vi "大富翁.vi"() -> ()   [LabVIEW 2014] (continued)
                n1038 = call "顏色轉數字.vi"("顏色數字"=w422) -> ("數字"=w425:dbl)  [unwired: 2 in]
                n1039 = case shown="1, Default" w425 {
                  tunnel: [w443 w444 w445 w446] -> w429
                  frame 1, Default {
                    n1040 = local read "玩家一財產"() -> (w443:dbl)
                  }
                  frame 2 {
                    n1041 = local read "玩家二財產"() -> (w444:dbl)
                  }
                  frame 3 {
                    n1042 = local read "玩家三財產"() -> (w445:dbl)
                  }
                  frame 4 {
                    n1043 = local read "玩家四財產"() -> (w446:dbl)
                  }
                }
                n1044 = call "走到地.vi"("房子數量"=w436, "自己的地?"=w437, "旅館數量"=w435, "編號"=w434, "走到人財產"=w433) -> ("走到人-?"=w432:dbl, "蓋第幾棟"=w430:dbl, "地主+?"=w428:dbl, "破產?"=w424:bool)
                n1045 = Subtract(x=w433, y=w432) -> (x-y=w431:dbl)
                n1046 = Add(x=w428, y=w429) -> (x+y=w426:dbl)
                n1047 = case shown="1, Default" w425 {
                  tunnel: w426 -> [w439 w440 w441 w442]
                  frame 1, Default {
                    n1048 = local write "玩家一財產"(w439) -> ()
                  }
                  frame 2 {
                    n1049 = local write "玩家二財產"(w440) -> ()
                  }
                  frame 3 {
                    n1050 = local write "玩家三財產"(w441) -> ()
                  }
                  frame 4 {
                    n1051 = local write "玩家四財產"(w442) -> ()
                  }
                }
                n1052 = case shown="8" w430 {
                  frame 0, Default {
                  }
                  frame 1 {
                    n1053 = flat-sequence {
                      frame #0 {
                        n1054 = local write "3房1"(TRUE ("1房1")) -> ()
                      }
                      frame #1 {
                        n1055 = property on="3房1" class="Bool (strict)"("Visible"=TRUE) -> ()  [unwired: 2 in, 2 out]
                      }
                    }
                  }
                  frame 2 {
                    n1056 = flat-sequence {
                      frame #0 {
                        n1057 = local write "3房2"(TRUE ("1房2")) -> ()
                      }
                      frame #1 {
                        n1058 = property on="3房2" class="Bool (strict)"("Visible"=TRUE ("1房2")) -> ()  [unwired: 2 in, 2 out]
                      }
                    }
                  }
                  frame 3 {
                    n1059 = flat-sequence {
                      frame #0 {
                        n1060 = local write "3房3"(TRUE) -> ()
                      }
                      frame #1 {
                        n1061 = property on="3房3" class="Bool (strict)"("Visible"=TRUE) -> ()  [unwired: 2 in, 2 out]
                      }
                    }
                  }
                  frame 4 {
                    n1062 = flat-sequence {
                      frame #0 {
                        n1063 = local write "3房4"(TRUE) -> ()
                      }
                      frame #1 {
                        n1064 = property on="3房4" class="Bool (strict)"("Visible"=TRUE) -> ()  [unwired: 2 in, 2 out]
                      }
                    }
                  }
                  frame 5 {
                    n1065 = flat-sequence {
                      frame #0 {
                        n1066 = local write "3旅1"(TRUE) -> ()
                      }
                      frame #1 {
                        n1067 = property on="3旅1" class="Bool (strict)"("Visible"=TRUE) -> ()  [unwired: 2 in, 2 out]
                      }
                    }
                  }
                  frame 6 {
                    n1068 = flat-sequence {
                      frame #0 {
                        n1069 = local write "3旅2"(TRUE) -> ()
                      }
                      frame #1 {
                        n1070 = property on="3旅2" class="Bool (strict)"("Visible"=TRUE) -> ()  [unwired: 2 in, 2 out]
                      }
                    }
                  }
                  frame 7 {
                    n1071 = flat-sequence {
                      frame #0 {
                        n1072 = local write "3旅3"(TRUE) -> ()
                      }
                      frame #1 {
                        n1073 = property on="3旅3" class="Bool (strict)"("Visible"=TRUE) -> ()  [unwired: 2 in, 2 out]
                      }
                    }
                  }
                  frame 8 {
                    n1074 = flat-sequence {
                      frame #0 {
                        n1075 = local write "3旅4"(TRUE) -> ()
                      }
                      frame #1 {
                        n1076 = property on="3旅4" class="Bool (strict)"("Visible"=TRUE) -> ()  [unwired: 2 in, 2 out]
                      }
                    }
                  }
                }
                n1077 = case shown="1, Default" w427 {
                  tunnel: w431 -> [w463 w464 w465 w466]
                  frame 1, Default {
                    n1078 = local write "玩家一財產"(w463) -> ()
                  }
                  frame 2 {
                    n1079 = local write "玩家二財產"(w464) -> ()
                  }
                  frame 3 {
                    n1080 = local write "玩家三財產"(w465) -> ()
                  }
                  frame 4 {
                    n1081 = local write "玩家四財產"(w466) -> ()
                  }
                }
              }
              frame True {
                # "無主地"
                n1082 = call "購買土地.vi"() -> ("確定 2"=w473:bool)  [unwired: 3 in]
                n1083 = case shown="True" w473 {
                  tunnel: w472 -> [_ w477]
                  frame False {
                    # "不買"
                  }
                  frame True {
                    # "要買"
                    n1084 = local read "換誰?"() -> (w478:dbl)
                    n1085 = case shown="4" w478 {
                      tunnel: [w505 w506 w507 w508] -> w476
                      frame 1, Default {
                        n1086 = local read "玩家一財產"() -> (w505:dbl)
                      }
                      frame 2 {
                        n1087 = local read "玩家二財產"() -> (w506:dbl)
                      }
                      frame 3 {
                        n1088 = local read "玩家三財產"() -> (w507:dbl)
                      }
                      frame 4 {
                        n1089 = local read "玩家四財產"() -> (w508:dbl)
                      }
                    }
                    n1090 = call "各種價格.vi"("Numeric"=w477) -> ("買空地"=w475:dbl)  [unwired: 4 in, 5 out]
                    n1091 = Greater Or Equal?(x=w476, y=w475) -> (x >= y?=w474:bool)
                    n1092 = case shown="True" w474 {
                      tunnel: w477 -> [_ w479]
                      frame False {
                        # "錢不夠"
                        n1093 = call "錢不夠.vi"() -> ()  [unwired: 4 in]
                      }
                      frame True {
                        # "錢夠"
                        n1094 = local read "換誰?"() -> (w480:dbl)
                        n1095 = case shown="3" w480 {
                          selector: w480 -> [w484 w490 w496 w502]
                          tunnel: w479 -> [w483 w489 w495 w501]
                          frame 1, Default {
                            # "誰買了地"
                            n1096 = call "各種價格.vi"("Numeric"=w483) -> ("買空地"=w482:dbl)  [unwired: 4 in, 5 out]
                            n1097 = local read "玩家一財產"() -> (w486:dbl)
                            n1098 = Subtract(x=w486, y=w482) -> (x-y=w485:dbl)
                            n1099 = local write "玩家一財產"(w485) -> ()
                            n1100 = call "數字轉顏色.vi"("數字"=w484) -> ("顏色數字"=w481:dbl)  [unwired: 2 in]
                            n1101 = local write "3台北市"(w481) -> ()
                            n1102 = local write "台北市所有"(w481) -> ()
                          }
                          frame 2 {
                            # "誰買了地"
                            n1103 = call "各種價格.vi"("Numeric"=w489) -> ("買空地"=w488:dbl)  [unwired: 4 in, 5 out]
                            n1104 = local read "玩家二財產"() -> (w492:dbl)
                            n1105 = Subtract(x=w492, y=w488) -> (x-y=w491:dbl)
                            n1106 = local write "玩家二財產"(w491) -> ()
                            n1107 = call "數字轉顏色.vi"("數字"=w490) -> ("顏色數字"=w487:dbl)  [unwired: 2 in]
                            n1108 = local write "3台北市"(w487) -> ()
                            n1109 = local write "台北市所有"(w487) -> ()
                          }
                          frame 3 {
                            # "誰買了地"
                            n1110 = local read "玩家三財產"() -> (w497:dbl)
                            n1111 = call "各種價格.vi"("Numeric"=w495) -> ("買空地"=w494:dbl)  [unwired: 4 in, 5 out]
                            n1112 = Subtract(x=w497, y=w494) -> (x-y=w498:dbl)
                            n1113 = call "數字轉顏色.vi"("數字"=w496) -> ("顏色數字"=w493:dbl)  [unwired: 2 in]
                            n1114 = local write "玩家三財產"(w498) -> ()
                            n1115 = local write "3台北市"(w493) -> ()
                            n1116 = local write "台北市所有"(w493) -> ()
                          }
                          frame 4 {
                            # "誰買了地"
                            n1117 = call "各種價格.vi"("Numeric"=w501) -> ("買空地"=w500:dbl)  [unwired: 4 in, 5 out]
                            n1118 = local read "玩家四財產"() -> (w504:dbl)
                            n1119 = Subtract(x=w504, y=w500) -> (x-y=w503:dbl)
                            n1120 = local write "玩家四財產"(w503) -> ()
                            n1121 = call "數字轉顏色.vi"("數字"=w502) -> ("顏色數字"=w499:dbl)  [unwired: 2 in]
                            n1122 = local write "3台北市"(w499) -> ()
                            n1123 = local write "台北市所有"(w499) -> ()
                          }
                        }
                      }
                    }
                  }
                }
              }
            }
          }
          frame 4 {
            n1124 = local read "基隆市所有"() -> (w509:u32)
            n1125 = Equal?(x=w509, y=u32 16777215) -> (x = y?=w512:bool)
            n1126 = case shown="True" w512 {
              tunnel: w511 -> [w535 w573]
              tunnel: [w525 FALSE] -> w510
              frame False {
                # "有主地"
                n1127 = local read "換誰?"() -> (w528:dbl)
                n1128 = local read "基隆市所有"() -> (w516:u32)
                n1129 = call "數字轉顏色.vi"("數字"=w528) -> ("顏色數字"=w539:dbl)  [unwired: 2 in]
                n1130 = case shown="4" w528 {
                  tunnel: [w568 w569 w570 w571] -> w534
                  frame 1, Default {
                    n1131 = local read "玩家一財產"() -> (w568:dbl)
                  }
                  frame 2 {
                    n1132 = local read "玩家二財產"() -> (w569:dbl)
                  }
                  frame 3 {
                    n1133 = local read "玩家三財產"() -> (w570:dbl)
                  }
                  frame 4 {
                    n1134 = local read "玩家四財產"() -> (w571:dbl)
                  }
                }
                n1135 = Equal?(x=w516, y=w539) -> (x = y?=w538:bool)
                n1136 = local read "基隆市所有"() -> (w515:u32)
                n1137 = local read "4旅4"() -> (w517:bool)
                n1138 = local read "4旅3"() -> (w518:bool)
                n1139 = local read "4旅2"() -> (w519:bool)
                n1140 = local read "4旅1"() -> (w520:bool)
                n1141 = local read "4房4"() -> (w521:bool)
                n1142 = local read "4房3"() -> (w522:bool)
                n1143 = local read "4房2"() -> (w523:bool)
                n1144 = local read "4房1"() -> (w524:bool)
                n1145 = call "房子數量.vi"("房子 1"=w524, "房子 2"=w523, "房子 3"=w522, "房子 4"=w521, "旅館 1"=w520, "旅館 2"=w519, "旅館 3"=w518, "旅館 4"=w517) -> ("房子數"=w537:dbl, "旅館數"=w536:dbl)  [unwired: 18 in]
                n1146 = call "顏色轉數字.vi"("顏色數字"=w515) -> ("數字"=w526:dbl)  [unwired: 2 in]
                n1147 = case shown="1, Default" w526 {
                  tunnel: [w544 w545 w546 w547] -> w530
                  frame 1, Default {
                    n1148 = local read "玩家一財產"() -> (w544:dbl)
                  }
                  frame 2 {
                    n1149 = local read "玩家二財產"() -> (w545:dbl)
                  }
                  frame 3 {
                    n1150 = local read "玩家三財產"() -> (w546:dbl)
                  }
                  frame 4 {
                    n1151 = local read "玩家四財產"() -> (w547:dbl)
                  }
                }
                n1152 = call "走到地.vi"("房子數量"=w537, "自己的地?"=w538, "旅館數量"=w536, "編號"=w535, "走到人財產"=w534) -> ("走到人-?"=w533:dbl, "蓋第幾棟"=w531:dbl, "地主+?"=w529:dbl, "破產?"=w525:bool)
                n1153 = Subtract(x=w534, y=w533) -> (x-y=w532:dbl)
                n1154 = Add(x=w529, y=w530) -> (x+y=w527:dbl)
                n1155 = case shown="1, Default" w526 {
                  tunnel: w527 -> [w540 w541 w542 w543]
                  frame 1, Default {
                    n1156 = local write "玩家一財產"(w540) -> ()
                  }
                  frame 2 {
                    n1157 = local write "玩家二財產"(w541) -> ()
                  }
                  frame 3 {
                    n1158 = local write "玩家三財產"(w542) -> ()
                  }
                  frame 4 {
                    n1159 = local write "玩家四財產"(w543) -> ()
                  }
                }
                n1160 = case shown="8" w531 {
                  frame 0, Default {
                  }
                  frame 1 {
                    n1161 = flat-sequence {
                      frame #0 {
                        n1162 = local write "4房1"(TRUE ("1房1")) -> ()
                      }
                      frame #1 {
                        n1163 = property on="4房1" class="Bool (strict)"("Visible"=TRUE) -> ()  [unwired: 2 in, 2 out]
                      }
                    }
                  }
                  frame 2 {
                    n1164 = flat-sequence {
                      frame #0 {
                        n1165 = local write "4房2"(TRUE ("1房2")) -> ()
                      }
                      frame #1 {
                        n1166 = property on="4房2" class="Bool (strict)"("Visible"=TRUE ("1房2")) -> ()  [unwired: 2 in, 2 out]
                      }
                    }
                  }
                  frame 3 {
                    n1167 = flat-sequence {
                      frame #0 {
                        n1168 = local write "4房3"(TRUE) -> ()
                      }
                      frame #1 {
                        n1169 = property on="4房3" class="Bool (strict)"("Visible"=TRUE) -> ()  [unwired: 2 in, 2 out]
                      }
                    }
                  }
                  frame 4 {
                    n1170 = flat-sequence {
                      frame #0 {
                        n1171 = local write "4房4"(TRUE) -> ()
                      }
                      frame #1 {
                        n1172 = property on="4房4" class="Bool (strict)"("Visible"=TRUE) -> ()  [unwired: 2 in, 2 out]
                      }
                    }
                  }
                  frame 5 {
                    n1173 = flat-sequence {
                      frame #0 {
                        n1174 = local write "4旅1"(TRUE) -> ()
                      }
                      frame #1 {
                        n1175 = property on="4旅1" class="Bool (strict)"("Visible"=TRUE) -> ()  [unwired: 2 in, 2 out]
                      }
                    }
                  }
                  frame 6 {
                    n1176 = flat-sequence {
                      frame #0 {
                        n1177 = local write "4旅2"(TRUE) -> ()
                      }
                      frame #1 {
                        n1178 = property on="4旅2" class="Bool (strict)"("Visible"=TRUE) -> ()  [unwired: 2 in, 2 out]
                      }
                    }
                  }
                  frame 7 {
                    n1179 = flat-sequence {
                      frame #0 {
                        n1180 = local write "4旅3"(TRUE) -> ()
                      }
                      frame #1 {
                        n1181 = property on="4旅3" class="Bool (strict)"("Visible"=TRUE) -> ()  [unwired: 2 in, 2 out]
                      }
                    }
                  }
                  frame 8 {
                    n1182 = flat-sequence {
                      frame #0 {
                        n1183 = local write "4旅4"(TRUE) -> ()
                      }
                      frame #1 {
                        n1184 = property on="4旅4" class="Bool (strict)"("Visible"=TRUE) -> ()  [unwired: 2 in, 2 out]
                      }
                    }
                  }
                }
                n1185 = case shown="1, Default" w528 {
                  tunnel: w532 -> [w564 w565 w566 w567]
                  frame 1, Default {
                    n1186 = local write "玩家一財產"(w564) -> ()
                  }
                  frame 2 {
                    n1187 = local write "玩家二財產"(w565) -> ()
                  }
                  frame 3 {
                    n1188 = local write "玩家三財產"(w566) -> ()
                  }
                  frame 4 {
                    n1189 = local write "玩家四財產"(w567) -> ()
                  }
                }
              }
              frame True {
                # "無主地"
                n1190 = call "購買土地.vi"() -> ("確定 2"=w574:bool)  [unwired: 3 in]
                n1191 = case shown="True" w574 {
                  tunnel: w573 -> [_ w578]
                  frame False {
                    # "不買"
                  }
                  frame True {
                    # "要買"
                    n1192 = local read "換誰?"() -> (w579:dbl)
                    n1193 = case shown="4" w579 {
                      tunnel: [w606 w607 w608 w609] -> w577
                      frame 1, Default {
                        n1194 = local read "玩家一財產"() -> (w606:dbl)
                      }
                      frame 2 {
                        n1195 = local read "玩家二財產"() -> (w607:dbl)
                      }
                      frame 3 {
                        n1196 = local read "玩家三財產"() -> (w608:dbl)
                      }
                      frame 4 {
                        n1197 = local read "玩家四財產"() -> (w609:dbl)
                      }
                    }
                    n1198 = call "各種價格.vi"("Numeric"=w578) -> ("買空地"=w576:dbl)  [unwired: 4 in, 5 out]
                    n1199 = Greater Or Equal?(x=w577, y=w576) -> (x >= y?=w575:bool)
                    n1200 = case shown="True" w575 {
                      tunnel: w578 -> [_ w580]
                      frame False {
                        # "錢不夠"
                        n1201 = call "錢不夠.vi"() -> ()  [unwired: 4 in]
                      }
                      frame True {
                        # "錢夠"
                        n1202 = local read "換誰?"() -> (w581:dbl)
                        n1203 = case shown="4" w581 {
                          selector: w581 -> [w585 w591 w597 w603]
                          tunnel: w580 -> [w584 w590 w596 w602]
                          frame 1, Default {
                            # "誰買了地"
                            n1204 = call "各種價格.vi"("Numeric"=w584) -> ("買空地"=w583:dbl)  [unwired: 4 in, 5 out]
                            n1205 = local read "玩家一財產"() -> (w587:dbl)
                            n1206 = Subtract(x=w587, y=w583) -> (x-y=w586:dbl)
                            n1207 = local write "玩家一財產"(w586) -> ()
                            n1208 = call "數字轉顏色.vi"("數字"=w585) -> ("顏色數字"=w582:dbl)  [unwired: 2 in]
                            n1209 = local write "4基隆市"(w582) -> ()
                            n1210 = local write "基隆市所有"(w582) -> ()
                          }
                          frame 2 {
                            # "誰買了地"
                            n1211 = call "各種價格.vi"("Numeric"=w590) -> ("買空地"=w589:dbl)  [unwired: 4 in, 5 out]
                            n1212 = local read "玩家二財產"() -> (w593:dbl)
                            n1213 = Subtract(x=w593, y=w589) -> (x-y=w592:dbl)
                            n1214 = local write "玩家二財產"(w592) -> ()
                            n1215 = call "數字轉顏色.vi"("數字"=w591) -> ("顏色數字"=w588:dbl)  [unwired: 2 in]
                            n1216 = local write "4基隆市"(w588) -> ()
                            n1217 = local write "基隆市所有"(w588) -> ()
                          }
                          frame 3 {
                            # "誰買了地"
                            n1218 = local read "玩家三財產"() -> (w598:dbl)
                            n1219 = call "各種價格.vi"("Numeric"=w596) -> ("買空地"=w595:dbl)  [unwired: 4 in, 5 out]
                            n1220 = Subtract(x=w598, y=w595) -> (x-y=w599:dbl)
                            n1221 = call "數字轉顏色.vi"("數字"=w597) -> ("顏色數字"=w594:dbl)  [unwired: 2 in]
                            n1222 = local write "玩家三財產"(w599) -> ()
                            n1223 = local write "4基隆市"(w594) -> ()
                            n1224 = local write "基隆市所有"(w594) -> ()
                          }
                          frame 4 {
                            # "誰買了地"
                            n1225 = call "各種價格.vi"("Numeric"=w602) -> ("買空地"=w601:dbl)  [unwired: 4 in, 5 out]
                            n1226 = local read "玩家四財產"() -> (w605:dbl)
                            n1227 = Subtract(x=w605, y=w601) -> (x-y=w604:dbl)
                            n1228 = local write "玩家四財產"(w604) -> ()
                            n1229 = call "數字轉顏色.vi"("數字"=w603) -> ("顏色數字"=w600:dbl)  [unwired: 2 in]
                            n1230 = local write "4基隆市"(w600) -> ()
                            n1231 = local write "基隆市所有"(w600) -> ()
                          }
                        }
                      }
                    }
                  }
                }
              }
            }
          }
          frame 5, 16, 28 {
            # "命運"
            n1232 = local read "白色恐怖?"() -> (w611:bool)
            n1233 = case shown="False" w611 {
              tunnel: [w613 FALSE] -> w610
              frame False {
                # "非白色恐怖"
                n1234 = Random Number (0-1)() -> (number: 0 to 1=w618:dbl)
                n1235 = Multiply(x=w618, y=100.0) -> (x*y=w614:dbl)
                n1236 = Less?(x=w614, y=2.0) -> (x < y?=w615:bool)
                n1237 = case shown="False" w615 {
                  tunnel: w614 -> [w620 _]
                  tunnel: [w619 w889] -> w613
                  frame False {
                    # "2~100"
                    n1238 = Less?(x=w620, y=5.0) -> (x < y?=w621:bool)
                    n1239 = case shown="False" w621 {
                      tunnel: w620 -> [w624 _]
                      tunnel: [w623 FALSE] -> w619
                      frame False {
                        # "5~100"
                        n1240 = Less?(x=w624, y=10.0) -> (x < y?=w625:bool)
                        n1241 = case shown="False" w625 {
                          tunnel: w624 -> [w628 _]
                          tunnel: [w627 FALSE] -> w623
                          frame False {
                            # "10~100"
                            n1242 = Less?(x=w628, y=30.0) -> (x < y?=w629:bool)
                            n1243 = case shown="False" w629 {
                              tunnel: w628 -> [w632 _]
                              tunnel: [w631 w822] -> w627
                              frame False {
                                # "30~100"
                                n1244 = Less?(x=w632, y=45.0) -> (x < y?=w633:bool)
                                n1245 = case shown="False" w633 {
                                tunnel: w632 -> [w636 _]
                                tunnel: [w635 w799] -> w631
                                frame False {
                                # "45~100"
                                n1246 = Less?(x=w636, y=54.0) -> (x < y?=w637:bool)
                                n1247 = case shown="False" w637 {
                                tunnel: w636 -> [w640 _]
                                tunnel: [w639 w776] -> w635
                                frame False {
                                # "54~100"
                                n1248 = Less?(x=w640, y=58.0) -> (x < y?=w641:bool)
                                n1249 = case shown="False" w641 {
                                tunnel: w640 -> [w644 _]
                                tunnel: [w643 w753] -> w639
                                frame False {
                                # "58~100"
                                n1250 = Less?(x=w644, y=60.0) -> (x < y?=w645:bool)
                                n1251 = case shown="False" w645 {
                                tunnel: w644 -> [w648 _]
                                tunnel: [w647 w728] -> w643
                                frame False {
                                # "58~60"
                                n1252 = Less?(x=w648, y=74.0) -> (x < y?=w649:bool)
                                n1253 = case shown="False" w649 {
                                tunnel: w648 -> [w652 _]
                                tunnel: [w651 FALSE] -> w647
                                frame False {
                                # "60~84"
                                n1254 = Less?(x=w652, y=84.0) -> (x < y?=w653:bool)
                                n1255 = case shown="False" w653 {
                                tunnel: w652 -> [w656 _]
                                tunnel: [w655 FALSE] -> w651
                                frame False {
                                # "84~94"
                                n1256 = Less?(x=w656, y=94.0) -> (x < y?=w657:bool)
                                n1257 = case shown="False" w657 {
                                tunnel: w656 -> [w660 _]
                                tunnel: [w659 FALSE] -> w655
                                frame False {
                                # "94~99"
                                n1258 = Less?(x=w660, y=99.0) -> (x < y?=w661:bool)
                                n1259 = case shown="False" w661 {
                                tunnel: w660 -> [_ _]
                                tunnel: [FALSE FALSE] -> w659
                                frame False {
                                n1260 = local read "玩家三財產"() -> (w667:dbl)
                                n1261 = local read "玩家四財產"() -> (w665:dbl)
                                n1262 = local read "玩家一財產"() -> (w671:dbl)
                                n1263 = local read "玩家二財產"() -> (w669:dbl)
                                n1264 = Add(x=w665, y=3000.0) -> (x+y=w664:dbl)
                                n1265 = Add(x=w671, y=3000.0) -> (x+y=w670:dbl)
                                n1266 = Add(x=w669, y=3000.0) -> (x+y=w668:dbl)
                                n1267 = Add(x=w667, y=3000.0) -> (x+y=w666:dbl)
                                n1268 = local write "玩家一財產"(w670) -> ()
                                n1269 = local write "玩家二財產"(w668) -> ()
                                n1270 = local write "玩家四財產"(w664) -> ()
                                n1271 = local write "玩家三財產"(w666) -> ()
                                n1272 = call "命運通通+3000.vi"() -> ()  [unwired: 4 in]
                                }
                                frame True {
                                n1273 = call "命運+3000.vi"() -> ()  [unwired: 4 in]
                                n1274 = local read "換誰?"() -> (w677:dbl)
                                n1275 = case shown="1, Default" w677 {
                                tunnel: [w685 w686 w687 w688] -> w678
                                frame 1, Default {
                                n1276 = local read "玩家一財產"() -> (w685:dbl)
                                }
                                frame 2 {
                                n1277 = local read "玩家二財產"() -> (w686:dbl)
                                }
                                frame 3 {
                                n1278 = local read "玩家三財產"() -> (w687:dbl)
                                }
                                frame 4 {
                                n1279 = local read "玩家四財產"() -> (w688:dbl)
                                }
                                }
                                n1280 = Add(x=w678, y=3000.0) -> (x+y=w680:dbl)
                                n1281 = case shown="1, Default" w677 {
                                tunnel: w680 -> [w681 w682 w683 w684]
                                frame 1, Default {
                                n1282 = local write "玩家一財產"(w681) -> ()
                                }
                                frame 2 {
                                n1283 = local write "玩家二財產"(w682) -> ()
                                }
                                frame 3 {
                                n1284 = local write "玩家三財產"(w683) -> ()
                                }
                                frame 4 {
                                n1285 = local write "玩家四財產"(w684) -> ()
                                }
                                }
                                }
                                }
                                }
                                frame True {
                                n1286 = call "命運+2000.vi"() -> ()  [unwired: 4 in]
                                n1287 = local read "換誰?"() -> (w690:dbl)
                                n1288 = case shown="1, Default" w690 {
                                tunnel: [w698 w699 w700 w701] -> w691
                                frame 1, Default {
                                n1289 = local read "玩家一財產"() -> (w698:dbl)
                                }
                                frame 2 {
                                n1290 = local read "玩家二財產"() -> (w699:dbl)
                                }
                                frame 3 {
                                n1291 = local read "玩家三財產"() -> (w700:dbl)
                                }
                                frame 4 {
                                n1292 = local read "玩家四財產"() -> (w701:dbl)
                                }
                                }
                                n1293 = Add(x=w691, y=2000.0) -> (x+y=w693:dbl)
                                n1294 = case shown="1, Default" w690 {
                                tunnel: w693 -> [w694 w695 w696 w697]
                                frame 1, Default {
                                n1295 = local write "玩家一財產"(w694) -> ()
                                }
                                frame 2 {
                                n1296 = local write "玩家二財產"(w695) -> ()
                                }
                                frame 3 {
                                n1297 = local write "玩家三財產"(w696) -> ()
                                }
                                frame 4 {
                                n1298 = local write "玩家四財產"(w697) -> ()
                                }
                                }
                                }
                                }
                                }
                                frame True {
                                n1299 = call "命運+1000.vi"() -> ()  [unwired: 4 in]
                                n1300 = local read "換誰?"() -> (w703:dbl)
                                n1301 = case shown="1, Default" w703 {
                                tunnel: [w711 w712 w713 w714] -> w704
                                frame 1, Default {
                                n1302 = local read "玩家一財產"() -> (w711:dbl)
                                }
                                frame 2 {
                                n1303 = local read "玩家二財產"() -> (w712:dbl)
                                }
                                frame 3 {
                                n1304 = local read "玩家三財產"() -> (w713:dbl)
                                }
                                frame 4 {
                                n1305 = local read "玩家四財產"() -> (w714:dbl)
                                }
                                }
                                n1306 = Add(x=w704, y=1000.0) -> (x+y=w706:dbl)
                                n1307 = case shown="1, Default" w703 {
                                tunnel: w706 -> [w707 w708 w709 w710]
                                frame 1, Default {
                                n1308 = local write "玩家一財產"(w707) -> ()
                                }
                                frame 2 {
                                n1309 = local write "玩家二財產"(w708) -> ()
                                }
                                frame 3 {
                                n1310 = local write "玩家三財產"(w709) -> ()
                                }
                                frame 4 {
                                n1311 = local write "玩家四財產"(w710) -> ()
                                }
                                }
                                }
                                }
                                }
                                frame True {
                                n1312 = local read "換誰?"() -> (w716:dbl)
                                n1313 = call "命運+500.vi"() -> ()  [unwired: 4 in]
                                n1314 = case shown="1, Default" w716 {
                                tunnel: [w724 w725 w726 w727] -> w717
                                frame 1, Default {
                                n1315 = local read "玩家一財產"() -> (w724:dbl)
                                }
                                frame 2 {
                                n1316 = local read "玩家二財產"() -> (w725:dbl)
                                }
                                frame 3 {
                                n1317 = local read "玩家三財產"() -> (w726:dbl)
                                }
                                frame 4 {
                                n1318 = local read "玩家四財產"() -> (w727:dbl)
                                }
                                }
                                n1319 = Add(x=w717, y=500.0) -> (x+y=w719:dbl)
                                n1320 = case shown="1, Default" w716 {
                                tunnel: w719 -> [w720 w721 w722 w723]
                                frame 1, Default {
                                n1321 = local write "玩家一財產"(w720) -> ()
                                }
                                frame 2 {
                                n1322 = local write "玩家二財產"(w721) -> ()
                                }
                                frame 3 {
                                n1323 = local write "玩家三財產"(w722) -> ()
                                }
                                frame 4 {
                                n1324 = local write "玩家四財產"(w723) -> ()
                                }
                                }
                                }
                                }
                                }
                                frame True {
                                # "58~60"
                                n1325 = stacked-sequence {
                                tunnel: [_ w741] -> w728
                                frame #0 {
                                n1326 = call "命運通通扣3000.vi"() -> ()  [unwired: 4 in]
                                n1327 = local read "玩家三財產"() -> (w732:dbl)
                                n1328 = local read "玩家二財產"() -> (w734:dbl)
                                n1329 = local read "玩家一財產"() -> (w736:dbl)
                                n1330 = Subtract(x=w732, y=3000.0) -> (x-y=w731:dbl)
                                n1331 = Subtract(x=w734, y=3000.0) -> (x-y=w733:dbl)
                                n1332 = local read "玩家四財產"() -> (w730:dbl)
                                n1333 = Subtract(x=w736, y=3000.0) -> (x-y=w735:dbl)
                                n1334 = Subtract(x=w730, y=3000.0) -> (x-y=w729:dbl)
                                n1335 = local write "玩家三財產"(w731) -> ()
                                n1336 = local write "玩家二財產"(w733) -> ()
                                n1337 = local write "玩家四財產"(w729) -> ()
                                n1338 = local write "玩家一財產"(w735) -> ()
                                }
                                frame #1 {
                                n1339 = local read "玩家四財產"() -> (w750:dbl)
                                n1340 = local read "玩家三財產"() -> (w749:dbl)
                                n1341 = local read "玩家二財產"() -> (w748:dbl)
                                n1342 = local read "玩家一財產"() -> (w747:dbl)
                                n1343 = Less Than 0?(x=w750) -> (x < 0?=w746:bool)
                                n1344 = Less Than 0?(x=w748) -> (x < 0?=w744:bool)
                                n1345 = Less Than 0?(x=w749) -> (x < 0?=w745:bool)
                                n1346 = Less Than 0?(x=w747) -> (x < 0?=w743:bool)
                                n1347 = Compound Arithmetic op=OR(w746, w745, w744, w743) -> (w742:bool)
                                n1348 = case shown="True" w742 {
                                tunnel: [FALSE TRUE] -> w741
                                frame False {
                                }
                                frame True {
                                n1349 = call "破產了.vi"() -> ()  [unwired: 4 in]
                                }
                                }
                                }
                                }
                                }
                                }
                                }
                                frame True {
                                # "54~58"
                                n1350 = stacked-sequence {
                                tunnel: [_ w766] -> w753
                                frame #0 {
                                n1351 = call "命運罰3000.vi"() -> ()  [unwired: 4 in]
                                n1352 = local read "換誰?"() -> (w754:dbl)
                                n1353 = case shown="1, Default" w754 {
                                tunnel: [w762 w763 w764 w765] -> w755
                                frame 1, Default {
                                n1354 = local read "玩家一財產"() -> (w762:dbl)
                                }
                                frame 2 {
                                n1355 = local read "玩家二財產"() -> (w763:dbl)
                                }
                                frame 3 {
                                n1356 = local read "玩家三財產"() -> (w764:dbl)
                                }
                                frame 4 {
                                n1357 = local read "玩家四財產"() -> (w765:dbl)
                                }
                                }
                                n1358 = Subtract(x=w755, y=3000.0) -> (x-y=w757:dbl)
                                n1359 = case shown="1, Default" w754 {
                                tunnel: w757 -> [w758 w759 w760 w761]
                                frame 1, Default {
                                n1360 = local write "玩家一財產"(w758) -> ()
                                }
                                frame 2 {
                                n1361 = local write "玩家二財產"(w759) -> ()
                                }
                                frame 3 {
                                n1362 = local write "玩家三財產"(w760) -> ()
                                }
                                frame 4 {
                                n1363 = local write "玩家四財產"(w761) -> ()
                                }
                                }
                                }
                                frame #1 {
                                n1364 = local read "換誰?"() -> (w768:dbl)
                                n1365 = case shown="1, Default" w768 {
                                tunnel: [w772 w773 w774 w775] -> w769
                                frame 1, Default {
                                n1366 = local read "玩家一財產"() -> (w772:dbl)
                                }
                                frame 2 {
                                n1367 = local read "玩家二財產"() -> (w773:dbl)
                                }
                                frame 3 {
                                n1368 = local read "玩家三財產"() -> (w774:dbl)
                                }
                                frame 4 {
                                n1369 = local read "玩家四財產"() -> (w775:dbl)
                                }
                                }
                                n1370 = Less Than 0?(x=w769) -> (x < 0?=w767:bool)
                                n1371 = case shown="True" w767 {
                                tunnel: [FALSE TRUE] -> w766
                                frame False {
                                }
                                frame True {
                                n1372 = call "破產了.vi"() -> ()  [unwired: 4 in]
                                }
                                }
                                }
                                }
                                }
                                }
                                }
                                frame True {
                                # "45~54"
                                n1373 = stacked-sequence {
                                tunnel: [_ w789] -> w776
                                frame #0 {
                                n1374 = call "命運罰2000.vi"() -> ()  [unwired: 4 in]
                                n1375 = local read "換誰?"() -> (w777:dbl)
                                n1376 = case shown="1, Default" w777 {
                                tunnel: [w785 w786 w787 w788] -> w778
                                frame 1, Default {
                                n1377 = local read "玩家一財產"() -> (w785:dbl)
                                }
                                frame 2 {
                                n1378 = local read "玩家二財產"() -> (w786:dbl)
                                }
                                frame 3 {
                                n1379 = local read "玩家三財產"() -> (w787:dbl)
                                }
                                frame 4 {
                                n1380 = local read "玩家四財產"() -> (w788:dbl)
                                }
                                }
                                n1381 = Subtract(x=w778, y=2000.0) -> (x-y=w780:dbl)
                                n1382 = case shown="1, Default" w777 {
                                tunnel: w780 -> [w781 w782 w783 w784]
                                frame 1, Default {
                                n1383 = local write "玩家一財產"(w781) -> ()
                                }
                                frame 2 {
                                n1384 = local write "玩家二財產"(w782) -> ()
                                }
                                frame 3 {
                                n1385 = local write "玩家三財產"(w783) -> ()
                                }
                                frame 4 {
                                n1386 = local write "玩家四財產"(w784) -> ()
                                }
                                }
                                }
                                frame #1 {
                                n1387 = local read "換誰?"() -> (w791:dbl)
                                n1388 = case shown="1, Default" w791 {
                                tunnel: [w795 w796 w797 w798] -> w792
                                frame 1, Default {
                                n1389 = local read "玩家一財產"() -> (w795:dbl)
                                }
                                frame 2 {
                                n1390 = local read "玩家二財產"() -> (w796:dbl)
                                }
                                frame 3 {
                                n1391 = local read "玩家三財產"() -> (w797:dbl)
                                }
                                frame 4 {
                                n1392 = local read "玩家四財產"() -> (w798:dbl)
                                }
                                }
                                n1393 = Less Than 0?(x=w792) -> (x < 0?=w790:bool)
                                n1394 = case shown="True" w790 {
                                tunnel: [FALSE TRUE] -> w789
                                frame False {
                                }
                                frame True {
                                n1395 = call "破產了.vi"() -> ()  [unwired: 4 in]
                                }
                                }
                                }
                                }
                                }
                                }
                                }
                                frame True {
                                # "30~45"
                                n1396 = stacked-sequence {
                                tunnel: [_ w812] -> w799
                                frame #0 {
                                n1397 = call "命運罰1000.vi"() -> ()  [unwired: 4 in]
                                n1398 = local read "換誰?"() -> (w800:dbl)
                                n1399 = case shown="1, Default" w800 {
                                tunnel: [w808 w809 w810 w811] -> w801
                                frame 1, Default {
                                n1400 = local read "玩家一財產"() -> (w808:dbl)
                                }
                                frame 2 {
                                n1401 = local read "玩家二財產"() -> (w809:dbl)
                                }
                                frame 3 {
                                n1402 = local read "玩家三財產"() -> (w810:dbl)
                                }
                                frame 4 {
                                n1403 = local read "玩家四財產"() -> (w811:dbl)
                                }
                                }
                                n1404 = Subtract(x=w801, y=1000.0) -> (x-y=w803:dbl)
                                n1405 = case shown="1, Default" w800 {
                                tunnel: w803 -> [w804 w805 w806 w807]
                                frame 1, Default {
                                n1406 = local write "玩家一財產"(w804) -> ()
                                }
                                frame 2 {
                                n1407 = local write "玩家二財產"(w805) -> ()
                                }
                                frame 3 {
                                n1408 = local write "玩家三財產"(w806) -> ()
                                }
                                frame 4 {
                                n1409 = local write "玩家四財產"(w807) -> ()
                                }
                                }
                                }
                                frame #1 {
                                n1410 = local read "換誰?"() -> (w814:dbl)
                                n1411 = case shown="1, Default" w814 {
                                tunnel: [w818 w819 w820 w821] -> w815
                                frame 1, Default {
                                n1412 = local read "玩家一財產"() -> (w818:dbl)
                                }
                                frame 2 {
                                n1413 = local read "玩家二財產"() -> (w819:dbl)
                                }
                                frame 3 {
                                n1414 = local read "玩家三財產"() -> (w820:dbl)
                                }
                                frame 4 {
                                n1415 = local read "玩家四財產"() -> (w821:dbl)
                                }
                                }
                                n1416 = Less Than 0?(x=w815) -> (x < 0?=w813:bool)
                                n1417 = case shown="True" w813 {
                                tunnel: [FALSE TRUE] -> w812
                                frame False {
                                }
                                frame True {
                                n1418 = call "破產了.vi"() -> ()  [unwired: 4 in]
                                }
                                }
                                }
                                }
                                }
                                }
                              }
                              frame True {
                                # "10~30"
                                n1419 = stacked-sequence {
                                tunnel: [_ w835] -> w822
                                frame #0 {
                                n1420 = local read "換誰?"() -> (w826:dbl)
                                n1421 = call "命運罰500.vi"() -> ()  [unwired: 4 in]
                                n1422 = case shown="1, Default" w826 {
                                tunnel: [w831 w832 w833 w834] -> w825
                                frame 1, Default {
                                n1423 = local read "玩家一財產"() -> (w831:dbl)
                                }
                                frame 2 {
                                n1424 = local read "玩家二財產"() -> (w832:dbl)
                                }
                                frame 3 {
                                n1425 = local read "玩家三財產"() -> (w833:dbl)
                                }
                                frame 4 {
                                n1426 = local read "玩家四財產"() -> (w834:dbl)
                                }
                                }
                                n1427 = Subtract(x=w825, y=500.0) -> (x-y=w823:dbl)
                                n1428 = case shown="4" w826 {
                                tunnel: w823 -> [w827 w828 w829 w830]
                                frame 1, Default {
                                n1429 = local write "玩家一財產"(w827) -> ()
                                }
                                frame 2 {
                                n1430 = local write "玩家二財產"(w828) -> ()
                                }
                                frame 3 {
                                n1431 = local write "玩家三財產"(w829) -> ()
                                }
                                frame 4 {
                                n1432 = local write "玩家四財產"(w830) -> ()
                                }
                                }
                                }
                                frame #1 {
                                n1433 = local read "換誰?"() -> (w837:dbl)
                                n1434 = case shown="1, Default" w837 {
                                tunnel: [w841 w842 w843 w844] -> w838
                                frame 1, Default {
                                n1435 = local read "玩家一財產"() -> (w841:dbl)
                                }
                                frame 2 {
                                n1436 = local read "玩家二財產"() -> (w842:dbl)
                                }
                                frame 3 {
                                n1437 = local read "玩家三財產"() -> (w843:dbl)
                                }
                                frame 4 {
                                n1438 = local read "玩家四財產"() -> (w844:dbl)
                                }
                                }
                                n1439 = Less Than 0?(x=w838) -> (x < 0?=w836:bool)
                                n1440 = case shown="True" w836 {
                                tunnel: [FALSE TRUE] -> w835
                                frame False {
                                }
                                frame True {
                                n1441 = call "破產了.vi"() -> ()  [unwired: 4 in]
                                }
                                }
                                }
                                }
                              }
                            }
                          }
                          frame True {
                            # "5~10%"
                            n1442 = local read "換誰?"() -> (w846:dbl)
                            n1443 = case shown="1" w846 {
                              frame 0, Default {
                              }
                              frame 1 {
                                n1444 = local write "剩幾天 1"(2.0 ("剩幾天 1")) -> ()
                                n1445 = local write "位置 1"(13.0 ("位置 1")) -> ()
                                n1446 = property on="入獄 1" class="Bool (strict)"("Visible"=TRUE) -> ()  [unwired: 2 in, 2 out]
                                n1447 = property on="P1 棋子" class="Bool (strict)"("Left"=1503 ("Position:Left"), "Top"=112 ("Position:Top")) -> ()  [unwired: 2 in, 2 out]
                              }
                              frame 2 {
                                n1448 = local write "位置 2"(13.0 ("位置 2")) -> ()
                                n1449 = local write "剩幾天 2"(2.0 ("剩幾天 2")) -> ()
                                n1450 = property on="入獄 2" class="Bool (strict)"("Visible"=TRUE) -> ()  [unwired: 2 in, 2 out]
